vi "SubVI - Receive Report File.vi"(11 "file path (use dialog)":path) -> (0 "error out":errorcluster)   [LabVIEW 2017]
panel:
  out "Array 2":u8[](array[numeric])
  out "Array":string[][](array[string])
  out "Progress ( % )":u8
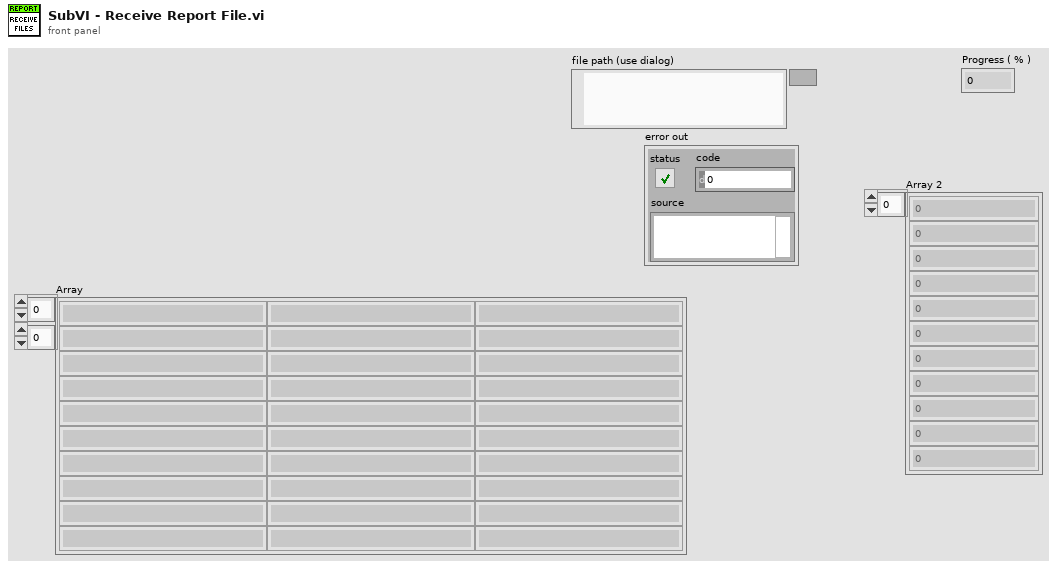
[diagram p1: front panel]
types:
  T1 = enum16{"open", "replace", "create", "open or create", "replace or create", "replace or create with confirmation"}
  T2 = enum16{"big-endian, network order", "native, host order", "little-endian"}
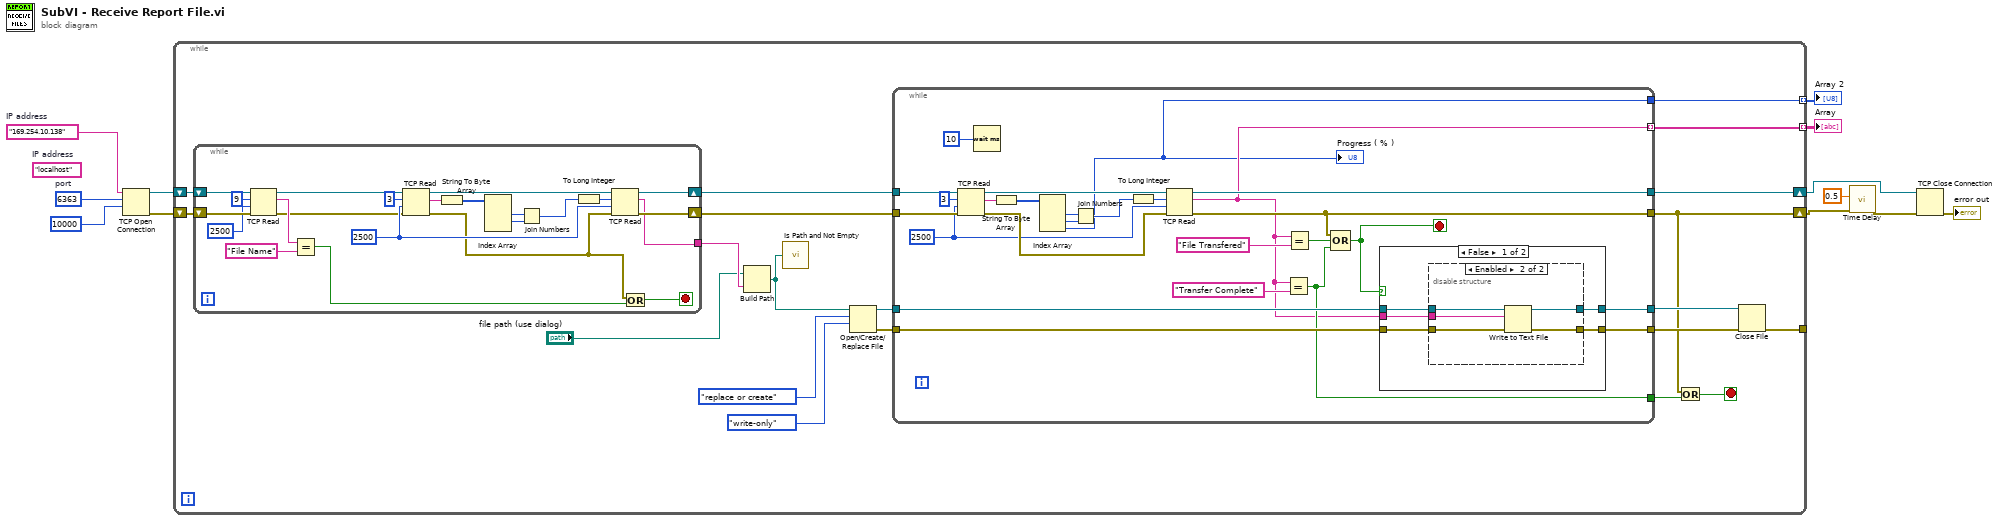
[diagram p0: block diagram]
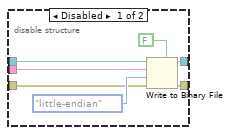
[diagram p2: hidden frame]
diagram:
  w2 = "169.254.10.138"  # IP address
  w12 = u16 6363  # port
  (unwired) "localhost"  # IP address
  n1 = TCP Open Connection(address=w2, remote port or service name=w12, timeout ms (60000)=10000 ("timeout ms (wait forever: -1)")) -> (connection ID=w10:refnum<k5>, error out=w9:errorcluster)  [unwired: 2 in]
  n2 = while {
    shift-right: [w20] -> w8
    shift-left: w10 -> [w26]
    shift-right: [w17] -> w7
    shift-left: w9 -> [w28]
    tunnel: [w16] -> w3 mode=indexing
    tunnel: [w14] -> _
    tunnel: [w13] -> w1 mode=indexing
    stop <- w18 stop-if-true
    n3 = while {
      shift-right: [w38] -> w27
      shift-left: w28 -> [w52]
      shift-right: [w39] -> w25
      shift-left: w26 -> [w51]
      tunnel: [w36] -> w24
      stop <- w35 stop-if-true
      w42 = 2500 ("timeout ms (25000)")
      n4 = TCP Read(connection ID=w51, bytes to read=9, error in (no error)=w52, 9:2500 ("timeout ms (25000)")) -> (connection ID out=w41:refnum<k5>, data out=w54:string, error out=w40:errorcluster)  [unwired: 1 in]
      n5 = Equal?(x=w54, y="File Name" ("data in")) -> (x = y?=w37:bool)
      n6 = TCP Read(connection ID=w41, bytes to read=3, error in (no error)=w40, 9:w42) -> (connection ID out=w45:refnum<k5>, data out=w49:string, error out=w34:errorcluster)  [unwired: 1 in]
      n7 = String To Byte Array(string=w49) -> (unsigned byte array=w48:u8[])
      n8 = Index Array(array=w48) -> (element #1=w47:u8, element #2=w46:u8)  [unwired: 3 in, 1 out]
      n9 = Join Numbers(hi=w47, lo=w46) -> ((hi.lo)=w43:u16)
      n10 = To Long Integer(number=w43) -> (32bit integer=w44:i32)
      n11 = TCP Read(connection ID=w45, bytes to read=w44, error in (no error)=w34, 9:w42) -> (connection ID out=w39:refnum<k5>, data out=w36:string, error out=w38:errorcluster)  [unwired: 1 in]
      n12 = Or(x=w34, y=w37) -> (x .or. y?=w35:bool)
    }
    n13 = Build Path(base path="file path (use dialog)", name or relative path=w24) -> (appended path=w15:path)
    n14 = call <vilib>:"Is Path and Not Empty.vi"("path"=w15) -> ()  [unwired: 4 in, 1 out]
    n15 = Open/Create/Replace File(file path (use dialog)=w15, operation (0:open)=T1."replace or create", access (0:read/write)=enum16{"read/write", "read-only", "write-only"}."write-only") -> (refnum out=w29:refnum<file>, error out=w30:errorcluster)  [unwired: 3 in, 1 out]
    n16 = while {
      tunnel: w25 -> [w81]
      tunnel: w27 -> [w80]
      tunnel: [w71] -> w20
      tunnel: [w58] -> w17
      tunnel: w30 -> [w69]
      tunnel: w29 -> [w68]
      tunnel: [w67] -> w21
      tunnel: [w66] -> w22
      tunnel: [w59] -> w19
      tunnel: [w57] -> w16 mode=indexing
      tunnel: [w56] -> w13
      stop <- w60 stop-if-true
      w63 = 2500 ("timeout ms (25000)")
      n17 = TCP Read(connection ID=w81, bytes to read=3, error in (no error)=w80, 9:w63) -> (connection ID out=w74:refnum<k5>, data out=w78:string, error out=w73:errorcluster)  [unwired: 1 in]
      n18 = Wait (ms)(milliseconds to wait=u32 10) -> ()  [unwired: 1 out]
      n19 = String To Byte Array(string=w78) -> (unsigned byte array=w77:u8[])
      n20 = Index Array(array=w77) -> (element #1=w76:u8, element #2=w75:u8, element #3=w56:u8)  [unwired: 3 in]
      "Progress ( % )" <- w56
      n21 = Join Numbers(hi=w76, lo=w75) -> ((hi.lo)=w64:u16)
      n22 = To Long Integer(number=w64) -> (32bit integer=w72:i32)
      n23 = TCP Read(connection ID=w74, bytes to read=w72, error in (no error)=w73, 9:w63) -> (connection ID out=w71:refnum<k5>, data out=w57:string, error out=w58:errorcluster)  [unwired: 1 in]
      n24 = Equal?(x=w57, y="Transfer Complete" ("data in")) -> (x = y?=w59:bool)
      n25 = Equal?(x=w57, y="File Transfered" ("data in")) -> (x = y?=w65:bool)
      n26 = Compound Arithmetic op=OR(w58, w65, w59) -> (w60:bool)
      n27 = case shown="False" w60 {
        tunnel: w69 -> [w86 w99]
        tunnel: w68 -> [w85 w100]
        tunnel: [w84 w100] -> w67
        tunnel: [w83 w99] -> w66
        tunnel: w57 -> [w82 _]
        frame False {
          n28 = disable-structure shown="Enabled" {
            disable-tunnel: w86 -> [w91 w97]
            disable-tunnel: w85 -> [w90 w98]
            disable-tunnel: [w89 w96] -> w84
            disable-tunnel: [w88 w95] -> w83
            disable-tunnel: w82 -> [w87 w94]
            frame Disabled {
              n29 = Write to Binary File(file (use dialog)=w90, data=w87, error in=w91, 5:FALSE ("prepend array or string size? (T)"), 9:T2."little-endian" ("byte order (0:big-endian, network order)")) -> (refnum out=w89:refnum<file>, error out=w88:errorcluster)  [unwired: 1 in, 1 out]
            }
            frame Enabled {
              n30 = Write to Text File(file (use dialog)=w98, text=w94, error in=w97) -> (refnum out=w96:refnum<file>, error out=w95:errorcluster)  [unwired: 1 in, 1 out]
            }
          }
        }
        frame True {
        }
      }
    }
    n31 = Or(x=w17, y=w19) -> (x .or. y?=w18:bool)
    n32 = Close File(refnum=w21, error in=w22) -> (error out=w14:errorcluster)  [unwired: 1 out]
  }
  "Array" <- w3
  "Array 2" <- w1
  n33 = call "Time Delay"("error in (no error)"=w7, "Delay Time (s)"=0.5) -> ("error out"=w6:errorcluster)  [unwired: 9 in]
  n34 = TCP Close Connection(connection ID=w8, error in (no error)=w6) -> (error out=→"error out":errorcluster)  [unwired: 1 in, 1 out]
